vi "generateShortCutMenu.vi"(8 "error in (no error)":errorcluster, 9 "activeRow?":bool, 10 "MenuRef":refnum<k9>, 11 "ScriptEditorV2 in":refnum<class "ScriptEditorV2.lvclass">) -> (0 "error out":errorcluster, 3 "ScriptEditorV2 out":refnum<class "ScriptEditorV2.lvclass">)   [LabVIEW 2011, in "Views.lvlib" / "ScriptEditor.lvlib" / "ScriptEditorV2.lvclass"]
uses:
  ScriptEditorV2.lvclass
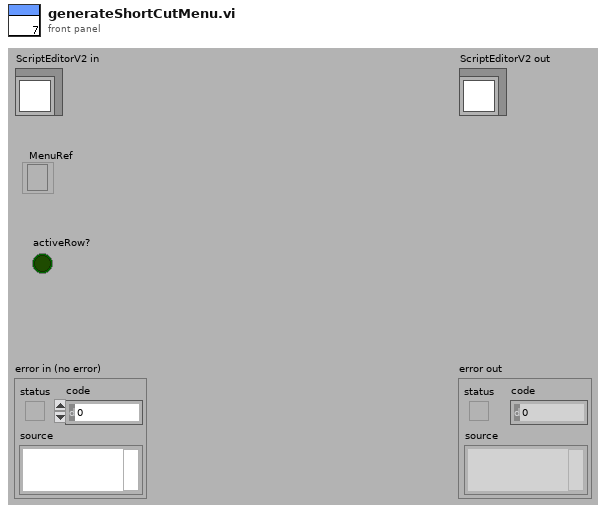
[diagram p1: front panel]
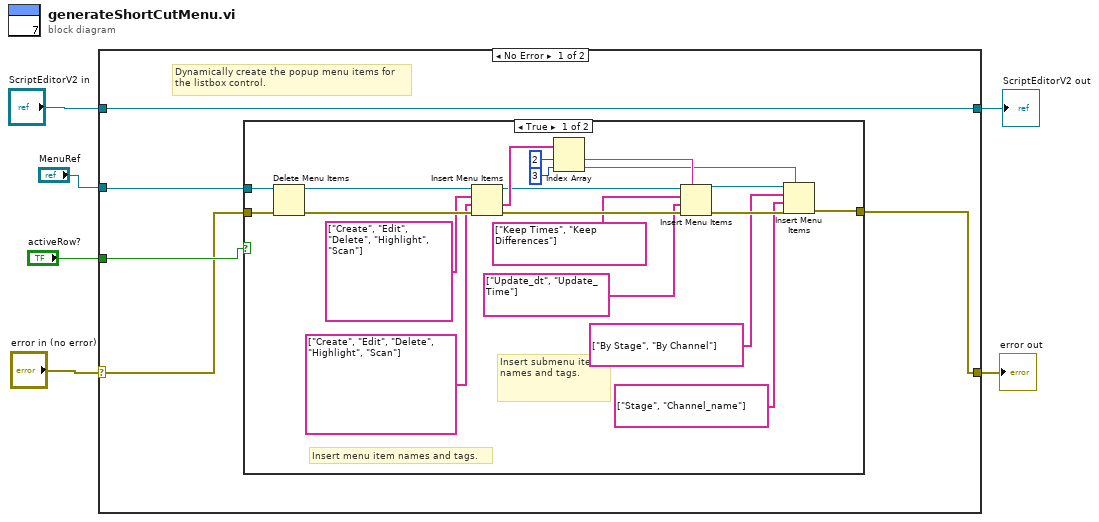
[diagram p0: block diagram]
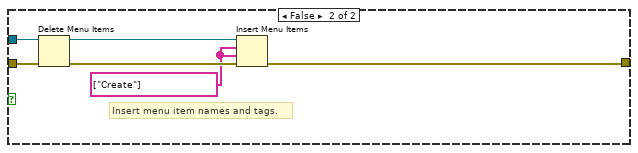
[diagram p2: hidden frame]
diagram:
  n1 = case shown="No Error" "error in (no error)" {
    selector: "error in (no error)" -> [w8 w39]
    tunnel: [w7 w39] -> w5
    tunnel: [w11 w38] -> w3
    tunnel: "ScriptEditorV2 in" -> [w11 w38]
    tunnel: "MenuRef" -> [w10 _]
    tunnel: "activeRow?" -> [w9 _]
    frame No Error {
      # "Dynamically create the popup menu items for the listbox control."
      n2 = case shown="True" w9 {
        tunnel: w10 -> [w20 w35]
        tunnel: w8 -> [w19 w34]
        tunnel: [w16 w33] -> w7
        frame True {
          # "Insert submenu item names and tags."
          # "Insert menu item names and tags."
          n3 = Delete Menu Items(6:w19, 9:w20) -> (0:w30:errorcluster, 3:w31:refnum<k9>)  [unwired: 2 in]
          n4 = Insert Menu Items(6:w30, 7:string[] ["Create", "Edit", "Delete", "Highlight", "Scan"], 8:string[] ["Create", "Edit", "Delete", "Highlight", "Scan"], 9:w31) -> (0:w24:errorcluster, 1:w27:string[], 3:w23:refnum<k9>)  [unwired: 2 in]
          n5 = Index Array(array=w27, index #1=2 ("index"), index #2=3) -> (element #1=w25:string, element #2=w14:string)
          n6 = Insert Menu Items(5:w25, 6:w24, 7:string[] ["Update_dt", "Update_Time"] ("item tags"), 8:string[] ["Keep Times", "Keep Differences"] ("item names"), 9:w23) -> (0:w17:errorcluster, 3:w18:refnum<k9>)  [unwired: 1 in, 1 out]
          n7 = Insert Menu Items(5:w14, 6:w17, 7:string[] ["Stage", "Channel_name"] ("item names"), 8:string[] ["By Stage", "By Channel"] ("item names"), 9:w18) -> (0:w16:errorcluster)  [unwired: 1 in, 2 out]
        }
        frame False {
          w32 = string[] ["Create"]
          # "Insert menu item names and tags."
          n8 = Delete Menu Items(6:w34, 9:w35) -> (0:w36:errorcluster, 3:w37:refnum<k9>)  [unwired: 2 in]
          n9 = Insert Menu Items(6:w36, 7:w32, 8:w32, 9:w37) -> (0:w33:errorcluster)  [unwired: 2 in, 2 out]
        }
      }
    }
    frame Error {
    }
  }
  "error out" <- w5
  "ScriptEditorV2 out" <- w3
